vi "RTD Read.vi"() -> ()   [LabVIEW 2018, in "Feed Module Engine.lvlib"]
uses:
  Feed Module Engine.lvlib
  <vilib>/DAQmx/read.llb/DAQmx Read (Analog Wfm 1Chan 1Samp).vi
  <vilib>/DAQmx/create/channels.llb/DAQmx Create Channel (AI-Temperature-RTD).vi
  <vilib>/DAQmx/miscellaneous.llb/DAQmx Fill In Error Info.vi
panel:
  in  "physical channels":tag="cDAQ2Mod4/ai0"
  in  "name to assign":string="Temp1"
  in  "units":i32(ring)=10143 items=["Deg C"=10143, "Deg F"=10144, "Kelvins"=10325, "Deg R"=10145, "From Custom Scale"=10065]
  in  "stop":bool
  out "data":waveform(dbl)
  out "Waveform Chart":waveform(dbl)(graph)
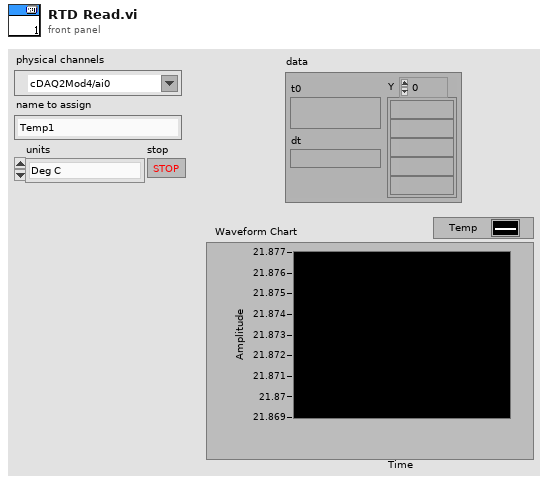
[diagram p1: front panel]
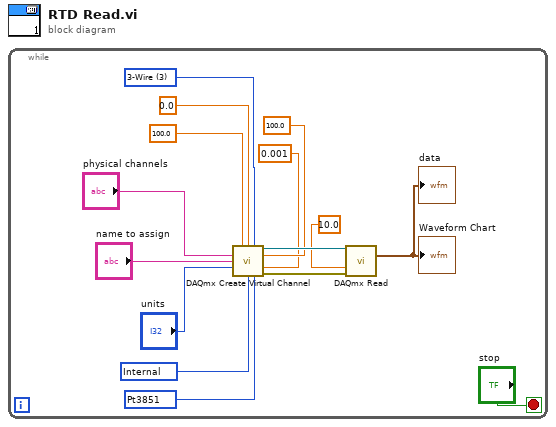
[diagram p0: block diagram]
diagram:
  n1 = while {
    stop <- "stop" stop-if-true
    w4 = 10200 items=["Internal"=10200, "External"=10167, "None"=10230] ("current excitation source")
    w8 = 10071 items=["Pt3750"=12481, "Pt3851"=10071, "Pt3911"=12482, "Pt3916"=10069, "Pt3920"=10053, "Pt3928"=12483, "Custom"=10137] ("rtd type")
    w9 = 3 items=["2-Wire"=2, "3-Wire"=3, "4-Wire"=4] ("resistance configuration")
    n2 = call-poly <vilib>:"DAQmx Create Virtual Channel.vi"("maximum value"=100.0, "minimum value"=0.0, "resistance configuration"=w9, "physical channels"="physical channels", "r0"=100.0, "name to assign"="name to assign", "units"="units", "current excitation value"=0.001, "current excitation source"=w4, "rtd type"=w8) -> ("task out"=w15:refnum<k21>, "error out"=w13:errorcluster)  [unwired: 4 in]
    n3 = call-poly <vilib>:"DAQmx Read.vi"("task/channels in"=w15, "timeout"=10.0, "error in"=w13) -> ("data"=→"data" →"Waveform Chart":waveform(dbl))  [unwired: 10 in, 2 out]
  }
